vi "Get BLISS_Get Image Lists.vi"(8 "error in":errorcluster, 11 "Data Parameters in":T1={"Start Time"=timestamp(3690155740.033191 s since 1904-01-01), "Save to Folder"=path "", "Forces in Theater"=[{"Force Commander"="BlissUT124", "Units"=[]}, {"Force Commander"="BlissMP146", "Units"=[]}, {"Force Commander"="BlissMP145", "Units"=[]}, {"Force Commander"="BlissMP140", "Units"=[]}, {"Force Commander"="BlissMP137", "Units"=[]}, {"Force Commander"="BlissMP135", "Units"=[]}, {"Force Commander"="BlissMP134", "Units"=[]}, {"Force Commander"="BlissMP132", "Units"=[]}, {"Force Commander"="BlissMA109", "Units"=[]}, {"Force Commander"="BlissMA107", "Units"=[]}, {"Force Commander"="BlissMA106", "Units"=[]}, {"Force Commander"="BlissMA101", "Units"=[]}, {"Force Commander"="BlissLU118", "Units"=[]}, {"Force Commander"="BlissLU117", "Units"=[]}, {"Force Commander"="BlissLU116", "Units"=[]}, {"Force Commander"="BlissLU115", "Units"=[]}, {"Force Commander"="BlissLU114", "Units"=[]}, {"Force Commander"="BlissLU113", "Units"=[]}, {"Force Commander"="BlissLU111", "Units"=[]}, {"Force Commander"="BlissLL185", "Units"=[]}, {"Force Commander"="BlissLL183", "Units"=[]}, {"Force Commander"="BlissLL173", "Units"=[]}, {"Force Commander"="BlissLL172", "Units"=[]}, {"Force Commander"="BlissLL171", "Units"=[]}, {"Force Commander"="BlissJH103", "Units"=[]}, {"Force Commander"="BlissJH102", "Units"=[]}, {"Force Commander"="BlissJH101", "Units"=[]}, {"Force Commander"="BlissJE116", "Units"=[]}, {"Force Commander"="BlissJE115", "Units"=[]}, {"Force Commander"="BlissJE114", "Units"=[]}, {"Force Commander"="BlissJE111", "Units"=[]}, {"Force Commander"="BlissHD183", "Units"=[]}, {"Force Commander"="BlissHD182", "Units"=[]}, {"Force Commander"="BlissHD181", "Units"=[]}, {"Force Commander"="BlissGPDFFPL", "Units"=[]}, {"Force Commander"="BlissEUWIPES", "Units"=[]}, {"Force Commander"="BlissEU179", "Units"=[]}, {"Force Commander"="BlissEU178", "Units"=[]}, {"Force Commander"="BlissEU177", "Units"=[]}, {"Force Commander"="Blissdvds02", "Units"=[]}, {"Force Commander"="BlissDOWIPES", "Units"=[]}, {"Force Commander"="BlissCR022", "Units"=[]}, {"Force Commander"="BlissCR021", "Units"=[]}, {"Force Commander"="BlissCG167", "Units"=[]}, {"Force Commander"="BlissCG166", "Units"=[]}, {"Force Commander"="BlissCG161", "Units"=[]}, {"Force Commander"="BlissCG160", "Units"=[]}, {"Force Commander"="BlissCG159", "Units"=[]}, {"Force Commander"="BlissCG158", "Units"=[]}, {"Force Commander"="BlissCG157", "Units"=[]}, {"Force Commander"="BlissCG156", "Units"=[]}, {"Force Commander"="BlissCG151", "Units"=[]}, {"Force Commander"="BlissCB172", "Units"=[]}, {"Force Commander"="BlissCB171", "Units"=[]}, {"Force Commander"="BlissCB108", "Units"=[]}, {"Force Commander"="BlissCB107", "Units"=[]}, {"Force Commander"="BlissBV181", "Units"=[]}, {"Force Commander"="BlissBV162", "Units"=[]}, {"Force Commander"="BlissAK177", "Units"=[]}, {"Force Commander"="BlissAK176", "Units"=[]}, {"Force Commander"="BlissAK175", "Units"=[]}, {"Force Commander"="BlissAK174", "Units"=[]}, {"Force Commander"="BlissAK173", "Units"=[]}, {"Force Commander"="BlissAK172", "Units"=[]}, {"Force Commander"="BlissAK171", "Units"=[]}, {"Force Commander"="BlissAK139", "Units"=[]}, {"Force Commander"="BlissAK134", "Units"=[]}, {"Force Commander"="BlissAK131", "Units"=[]}, {"Force Commander"="BlissAH163", "Units"=[]}, {"Force Commander"="BlissAH162", "Units"=[]}, {"Force Commander"="BlissAH161", "Units"=[]}, {"Force Commander"="BlissAH122", "Units"=[]}, {"Force Commander"="BlissAH121", "Units"=[]}, {"Force Commander"="BlissAD106", "Units"=[]}, {"Force Commander"="BlissAD104", "Units"=[]}, {"Force Commander"="BlissAB105", "Units"=[]}, {"Force Commander"="BlissAB104", "Units"=[]}]}) -> (0 "error out":errorcluster, 3 "Data Parameters out":T1={"Start Time"=timestamp(3690155740.033191 s since 1904-01-01), "Save to Folder"=path "D:/One Drive PG/Procter and Gamble/Varghese, Jacob - Deep Learning Vision System/Front Ear Foldover/BLISS Rejects (only R325 + R326) - not reviewed", "Forces in Theater"=[{"Force Commander"="BlissUT124", "Units"=[]}, {"Force Commander"="BlissMP146", "Units"=[]}, {"Force Commander"="BlissMP145", "Units"=[]}, {"Force Commander"="BlissMP140", "Units"=[]}, {"Force Commander"="BlissMP137", "Units"=[]}, {"Force Commander"="BlissMP135", "Units"=[]}, {"Force Commander"="BlissMP134", "Units"=[]}, {"Force Commander"="BlissMP132", "Units"=[]}, {"Force Commander"="BlissMA109", "Units"=[]}, {"Force Commander"="BlissMA107", "Units"=[]}, {"Force Commander"="BlissMA106", "Units"=[]}, {"Force Commander"="BlissMA101", "Units"=[]}, {"Force Commander"="BlissLU118", "Units"=[]}, {"Force Commander"="BlissLU117", "Units"=[]}, {"Force Commander"="BlissLU116", "Units"=[]}, {"Force Commander"="BlissLU115", "Units"=[]}, {"Force Commander"="BlissLU114", "Units"=[]}, {"Force Commander"="BlissLU113", "Units"=[]}, {"Force Commander"="BlissLU111", "Units"=[]}, {"Force Commander"="BlissLL185", "Units"=[]}, {"Force Commander"="BlissLL183", "Units"=[]}, {"Force Commander"="BlissLL173", "Units"=[]}, {"Force Commander"="BlissLL172", "Units"=[]}, {"Force Commander"="BlissLL171", "Units"=[]}, {"Force Commander"="BlissJH103", "Units"=[]}, {"Force Commander"="BlissJH102", "Units"=[]}, {"Force Commander"="BlissJH101", "Units"=[]}, {"Force Commander"="BlissJE116", "Units"=[]}, {"Force Commander"="BlissJE115", "Units"=[]}, {"Force Commander"="BlissJE114", "Units"=[]}, {"Force Commander"="BlissJE111", "Units"=[]}, {"Force Commander"="BlissHD183", "Units"=[]}, {"Force Commander"="BlissHD182", "Units"=[]}, {"Force Commander"="BlissHD181", "Units"=[]}, {"Force Commander"="BlissGPDFFPL", "Units"=[]}, {"Force Commander"="BlissEUWIPES", "Units"=[]}, {"Force Commander"="BlissEU179", "Units"=[]}, {"Force Commander"="BlissEU178", "Units"=[]}, {"Force Commander"="BlissEU177", "Units"=[]}, {"Force Commander"="Blissdvds02", "Units"=[]}, {"Force Commander"="BlissDOWIPES", "Units"=[]}, {"Force Commander"="BlissCR022", "Units"=[]}, {"Force Commander"="BlissCR021", "Units"=[]}, {"Force Commander"="BlissCG167", "Units"=[]}, {"Force Commander"="BlissCG166", "Units"=[]}, {"Force Commander"="BlissCG161", "Units"=[]}, {"Force Commander"="BlissCG160", "Units"=[]}, {"Force Commander"="BlissCG159", "Units"=[]}, {"Force Commander"="BlissCG158", "Units"=[]}, {"Force Commander"="BlissCG157", "Units"=[]}, {"Force Commander"="BlissCG156", "Units"=[]}, {"Force Commander"="BlissCG151", "Units"=[]}, {"Force Commander"="BlissCB172", "Units"=[]}, {"Force Commander"="BlissCB171", "Units"=[]}, {"Force Commander"="BlissCB108", "Units"=[]}, {"Force Commander"="BlissCB107", "Units"=[]}, {"Force Commander"="BlissBV181", "Units"=[]}, {"Force Commander"="BlissBV162", "Units"=[]}, {"Force Commander"="BlissAK177", "Units"=[]}, {"Force Commander"="BlissAK176", "Units"=[]}, {"Force Commander"="BlissAK175", "Units"=[]}, {"Force Commander"="BlissAK174", "Units"=[]}, {"Force Commander"="BlissAK173", "Units"=[]}, {"Force Commander"="BlissAK172", "Units"=[]}, {"Force Commander"="BlissAK171", "Units"=[]}, {"Force Commander"="BlissAK139", "Units"=[]}, {"Force Commander"="BlissAK134", "Units"=[]}, {"Force Commander"="BlissAK131", "Units"=[]}, {"Force Commander"="BlissAH163", "Units"=[]}, {"Force Commander"="BlissAH162", "Units"=[]}, {"Force Commander"="BlissAH161", "Units"=[]}, {"Force Commander"="BlissAH122", "Units"=[]}, {"Force Commander"="BlissAH121", "Units"=[]}, {"Force Commander"="BlissAD106", "Units"=[]}, {"Force Commander"="BlissAD104", "Units"=[]}, {"Force Commander"="BlissAB105", "Units"=[]}, {"Force Commander"="BlissAB104", "Units"=[]}]})   [LabVIEW 2020]
uses:
  MC5e Gobal_Variables.vi
  MC5e Squad_Info.ctl
  MC5e Unit_Status_List.ctl
  MC5e Data_Parameters.ctl
  MC5e Terrain types.ctl
  Location.ctl
  MC5e Unit.ctl
  MC5e Force.ctl
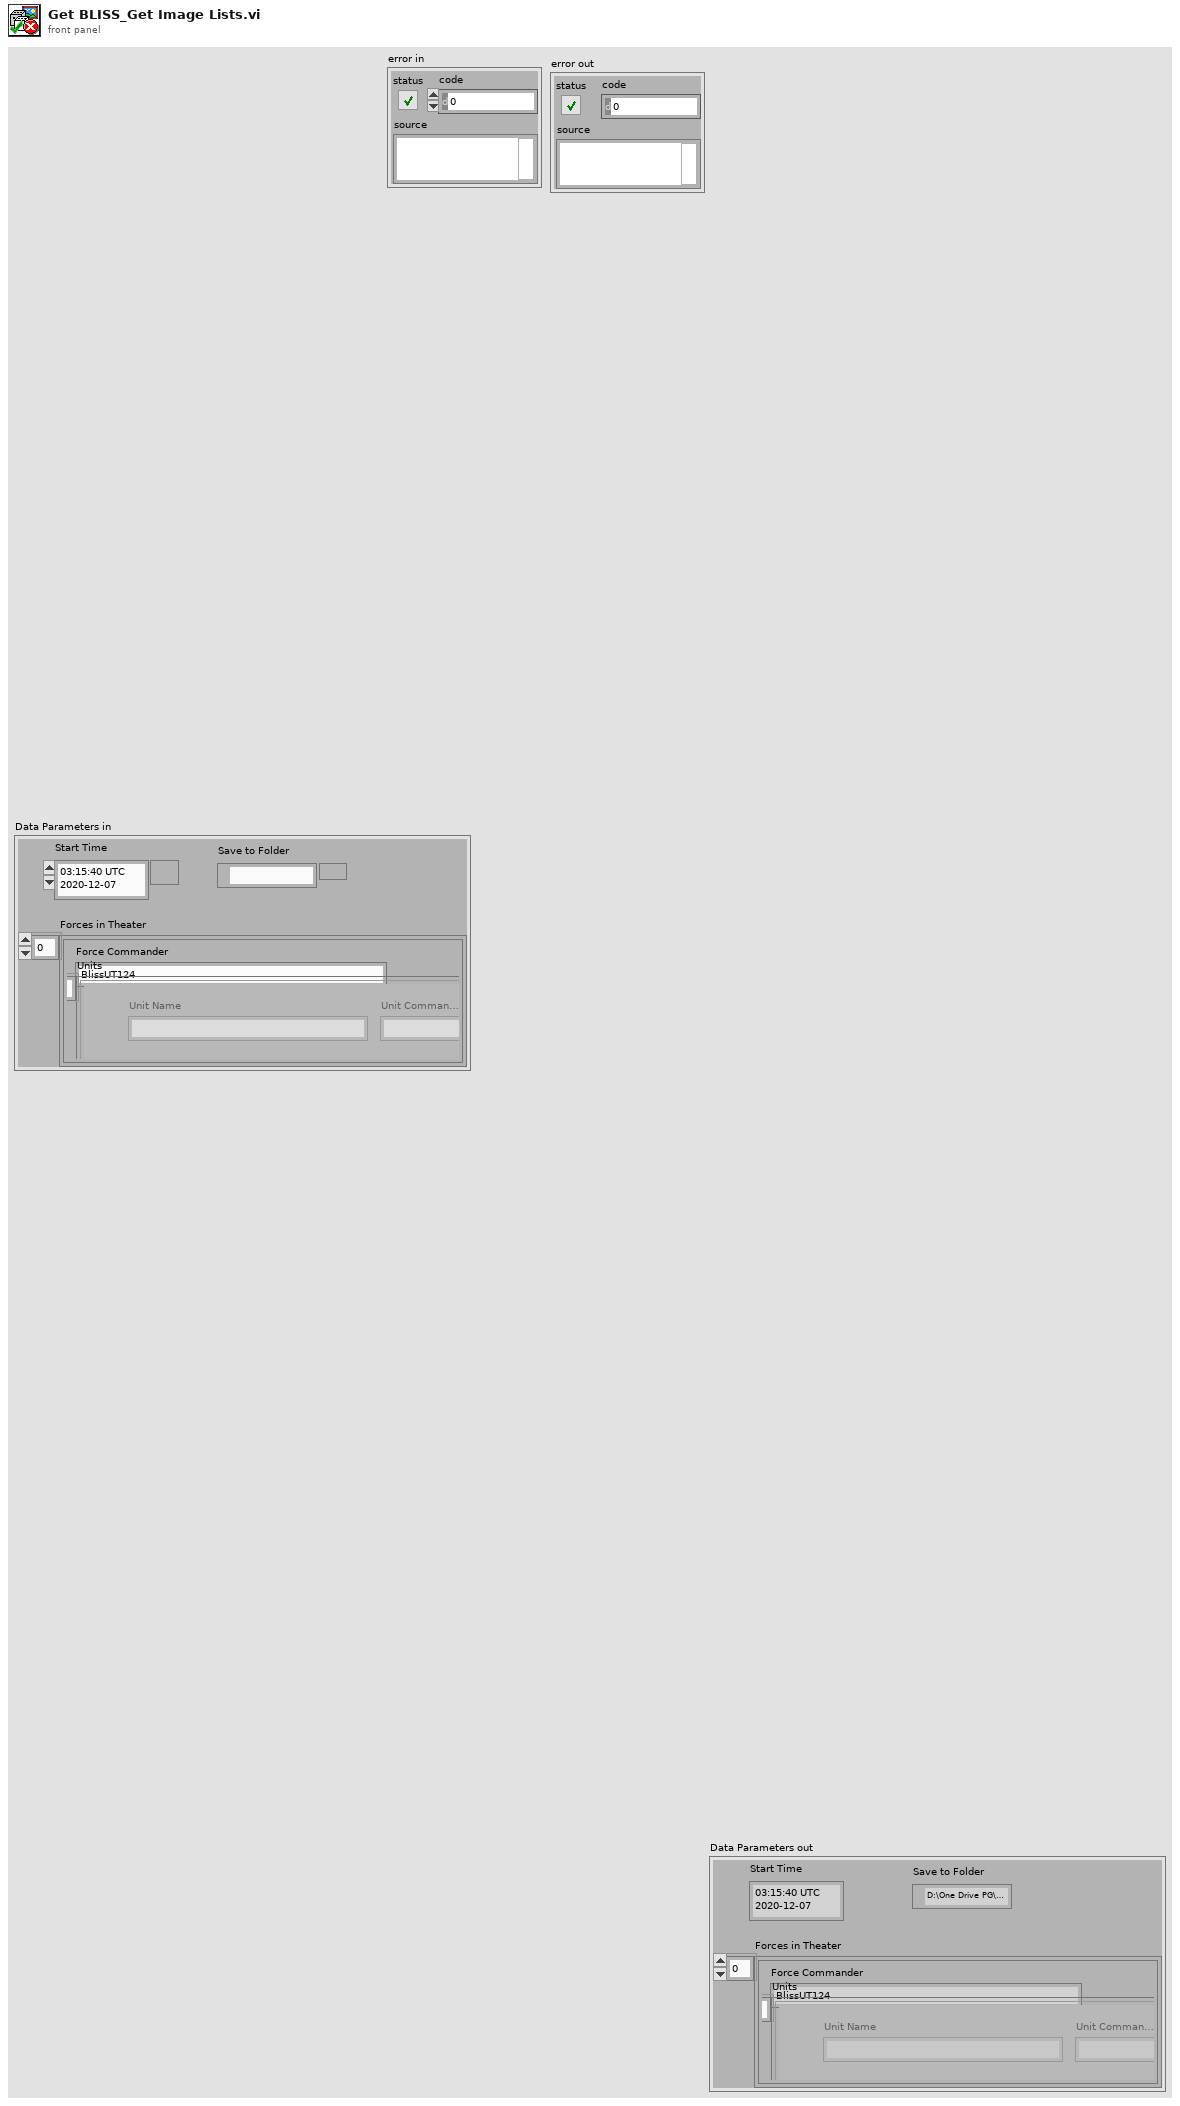
[diagram p1: front panel]
types:
  T1 = typedef "MC5e Data_Parameters.ctl" = cluster{"Start Time":timestamp, "Save to Folder":path, "Forces in Theater":T2[]}
  T2 = typedef "MC5e Force.ctl" = cluster{"Force Commander":string, "Units":T3[]}
  T3 = typedef "MC5e Unit.ctl" = cluster{"Squad List":T4, "Unit Fatigue Level":enum16{"Not Fatigued", "Fatigued", "Seriously Fatigued"}, "Flying Unit":bool, "Mounted Unit":bool, "Difficult Terrain Types":T6, "Full BR":dbl, "Defending from Stronghold":bool, "Speed":dbl, "Capacity %":dbl, "Morale":dbl, "Current BR":dbl, "Location":T7, "Unit Name":string, "Unit Commander":string, "Unit Notes":string}
  T4 = typedef "MC5e Unit_Status_List.ctl" = T5[]
  T5 = typedef "MC5e Squad_Info.ctl" = cluster{"Squad Name":string, "# Soldiers":dbl, "Battle Rating":dbl, "Flying":bool, "Mounted":bool, "Speed":dbl, "Range":dbl, "Morale":dbl, "Token Image":variant, "Max Endurance":dbl, "Current Endurance":dbl, "Difficult Terrain":T6}
  T6 = typedef "MC5e Terrain types.ctl" = cluster{"Artic / snow / ice)":bool, "Coast":bool, "Desert / sand":bool, "Forest / woodland":bool, "Grassland / plains":bool, "Mountain / canyons":bool, "Underdark / caverns":bool, "Acquatic / rivers, lakes, ocean":bool}
  T7 = typedef "Location.ctl" = cluster{"X coordinate":dbl, "Y coordinate":dbl}
  T8 = enum16{"Get Only Reject Images", "Get Only PBQA Images", "Get Both PBQA And Reject Images"}
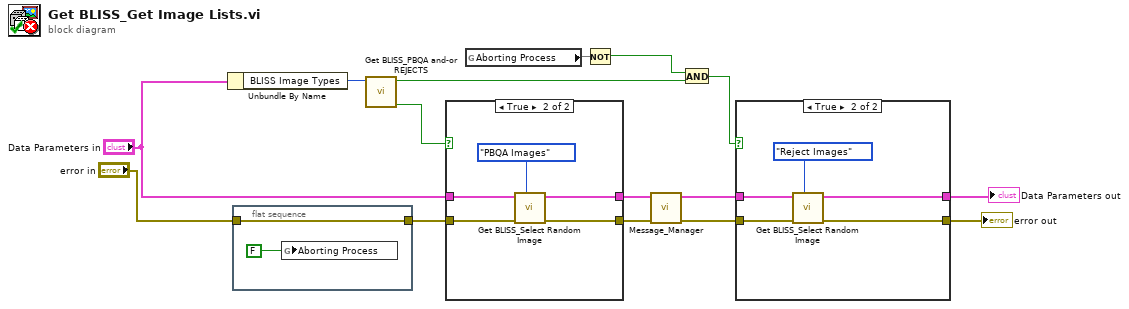
[diagram p0: block diagram]
diagram:
  n1 = Unbundle By Name("Data Parameters in") -> ("BLISS Image Types"=w14:T8)
  n2 = flat-sequence {
    tunnel: [w15] -> w10
    tunnel: "error in" -> [w15]
    frame #0 {
      n3 = global write "MC5e Gobal_Variables.vi" "Aborting Process"(FALSE ("Aborting Process")) -> ()
    }
  }
  n4 = call "Get BLISS_PBQA and-or REJECTS.vi"("BLISS Image Types"=w14) -> ("Get PBQA"=w13:bool, "Get Rejects"=w2:bool)  [unwired: 9 in]
  n5 = case shown="True" w13 {
    tunnel: w10 -> [w18 w23]
    tunnel: [w18 w22] -> w11
    tunnel: "Data Parameters in" -> [w17 w20]
    tunnel: [w17 w19] -> w6
    frame False {
    }
    frame True {
      n6 = call "Get BLISS_Select Random Image.vi"("BLISS Type"=enum16{"Reject Images", "PBQA Images"}."PBQA Images", "error in"=w23, "Data Parameters in"=w20) -> ("error out"=w22:errorcluster, "Data Parameters out"=w19:T1)  [unwired: 7 in]
    }
  }
  n7 = global read "MC5e Gobal_Variables.vi" "Aborting Process"() -> (w4)
  n8 = Not(x=w4) -> (.not. x?=w1:bool)
  n9 = call "Message_Manager.vi"("error in"=w11) -> ("error out"=w9:errorcluster)  [unwired: 5 in, 5 out]
  n10 = And(x=w1, y=w2) -> (x .and. y?=w3:bool)
  n11 = case shown="True" w3 {
    tunnel: [w25 w30] -> w12
    tunnel: w9 -> [w25 w28]
    tunnel: w6 -> [w24 w27]
    tunnel: [w24 w26] -> w5
    frame False {
    }
    frame True {
      n12 = call "Get BLISS_Select Random Image.vi"("BLISS Type"=enum16{"Reject Images", "PBQA Images"}."Reject Images", "error in"=w28, "Data Parameters in"=w27) -> ("error out"=w30:errorcluster, "Data Parameters out"=w26:T1)  [unwired: 7 in]
    }
  }
  "error out" <- w12
  "Data Parameters out" <- w5
